vi "Post-Bury.vi"(6 "Search Path":path[](array[path]), 8 "Error In":errorcluster, 10 "Grave In":refnum<vi>, 11 "VI In":refnum<vi>) -> (0 "Error Out":errorcluster, 2 "Grave Out":refnum<vi>, 3 "VI Out":refnum<vi>)   [LabVIEW 2018, in "Toolkit.lvlib"]
uses:
  Toolkit.lvlib
  Typedefs/Hooks.ctl
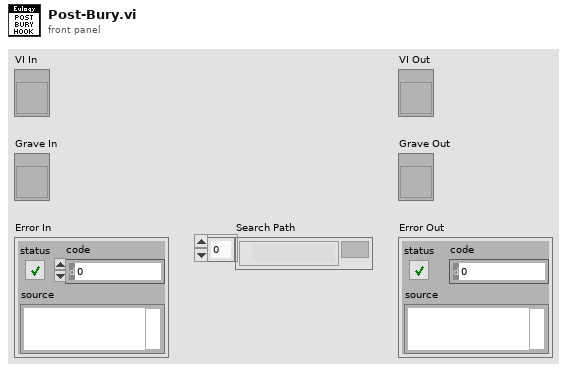
[diagram p1: front panel]
types:
  T1 = typedef "Toolkit.lvlib/Hooks.ctl" = enum16{"Pre-Bury", "Post-Bury", "Pre-Dig", "Post-Dig", "Pre-Reanimate", "Post-Reanimate", "Pre-Smite", "Post-Smite"}
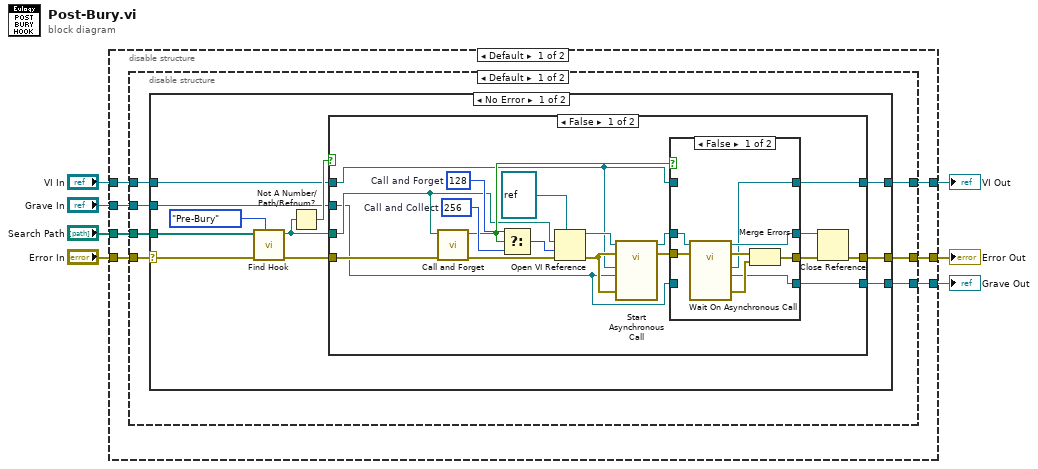
[diagram p0: block diagram]
diagram:
  n1 = disable-structure "Conditional Disable Structure" shown="Default" {
    disable-tunnel: "Error In" -> [w13 w74]
    disable-tunnel: "Search Path" -> [w12 _]
    disable-tunnel: "Grave In" -> [w11 w73]
    disable-tunnel: [w10 w73] -> w4
    disable-tunnel: "VI In" -> [w9 w75]
    disable-tunnel: [w8 w75] -> w2
    disable-tunnel: [w14 w74] -> w1
    frame condition #0 (active) {
      n2 = disable-structure "Conditional Disable Structure" shown="Default" {
        disable-tunnel: [w21 w70] -> w14
        disable-tunnel: w13 -> [w20 w70]
        disable-tunnel: w12 -> [w19 _]
        disable-tunnel: w11 -> [w18 w71]
        disable-tunnel: [w17 w71] -> w10
        disable-tunnel: w9 -> [w16 w72]
        disable-tunnel: [w15 w72] -> w8
        frame condition #0 (active) {
          n3 = case shown="No Error" w20 {
            selector: w20 -> [w30 w69]
            tunnel: [w31 w69] -> w21
            tunnel: w19 -> [w23 _]
            tunnel: w18 -> [w27 w68]
            tunnel: [w26 w68] -> w17
            tunnel: w16 -> [w25 w67]
            tunnel: [w24 w67] -> w15
            frame No Error {
              n4 = call "Find Hook.vi"("Hook"=Hooks."Pre-Bury", "Error In"=w30, "Search Path"=w23) -> ("Error Out"=w32:errorcluster, "Hook"=w29:path)  [unwired: 7 in]
              n5 = Not A Number/Path/Refnum?(number/path/refnum=w29) -> (NaN/Path/Refnum?=w28:bool)
              n6 = case shown="False" w28 {
                tunnel: w29 -> [w39 _]
                tunnel: w32 -> [w43 w66]
                tunnel: [w51 w66] -> w31
                tunnel: w27 -> [w35 w65]
                tunnel: [w38 w65] -> w26
                tunnel: w25 -> [w34 w64]
                tunnel: [w33 w64] -> w24
                frame False {
                  w45 = 256  # Call and Collect
                  w46 = 128  # Call and Forget
                  n7 = call "Call and Forget.vi"("Error In"=w43, "Hook"=w39) -> ("Error Out"=w42:errorcluster, "Call and Forget"=w41:bool)  [unwired: 8 in]
                  n8 = Select(t=w46, s=w41, f=w45) -> (s? t:f=w44:i32)
                  n9 = Open VI Reference(type specifier VI Refnum (for type only)=refnum<vi> refnum, vi path=w39, options=w44, error in (no error)=w42) -> (vi reference=w36:refnum<vi>, error out=w40:errorcluster)  [unwired: 2 in]
                  n10 = call-by-ref "Start Asynchronous Call"(reference=w36, error in=w40, "Error In"=w40, "Grave In"=w35, "VI In"=w34) -> (reference out=w50:refnum<vi>, error out=w48:errorcluster)  [unwired: 6 in, 3 out]
                  n11 = case shown="False" w41 {
                    tunnel: w50 -> [w59 w63]
                    tunnel: [w58 w63] -> w49
                    tunnel: w48 -> [w57 w62]
                    tunnel: [w55 w62] -> w47
                    tunnel: w35 -> [_ w61]
                    tunnel: [w53 w61] -> w38
                    tunnel: w34 -> [_ w60]
                    tunnel: [w52 w60] -> w33
                    frame False {
                      n12 = call-by-ref "Wait On Asynchronous Call"(reference=w59, error in=w57) -> (reference out=w58:refnum<vi>, error out=w56:errorcluster, "Error Out"=w54:errorcluster, "Grave Out"=w53:refnum<vi>, "VI Out"=w52:refnum<vi>)  [unwired: 9 in]
                      n13 = Merge Errors(w56, w54) -> (w55:errorcluster)
                    }
                    frame True {
                    }
                  }
                  n14 = Close Reference(reference=w49, error in (no error)=w47) -> (error out=w51:errorcluster)
                }
                frame True {
                }
              }
            }
            frame Error {
            }
          }
        }
        frame condition #1 {
        }
      }
    }
    frame condition #1 {
    }
  }
  "Error Out" <- w1
  "Grave Out" <- w4
  "VI Out" <- w2
